vi "ColorText Facade.vi"(0 "Data In":T4, 2 "Display State In":T2, 3 "Container State":T3) -> (6 "Data Out":T4, 7 "Display State Out":T2, 8 "Action":T1)   [LabVIEW 2020, in "Code.xctl"]
uses:
  Code.xctl
  ColorText Data.ctl
  <vilib>/_xctls/Container State.ctl
  ColorText State.ctl
  <vilib>/_xctls/Action.ctl
  <vilib>/_xctls/XControlSupport.lvlib
panel:
  in  "Rows":string
  in  "Code":string
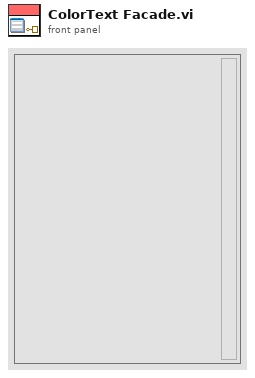
[diagram p1: front panel]
types:
  T1 = typedef "XControlSupport.lvlib/Action.ctl" = cluster{"Data Changed?":bool, "State Changed?":bool, "Action Name":string}
  T2 = typedef "Code.xctl/ColorText State.ctl" = cluster{"Numeric":dbl}
  T3 = typedef "XControlSupport.lvlib/Container State.ctl" = cluster{"Indicator?":bool, "Run Mode?":bool, " Refnum":refnum<vi>}
  T4 = typedef "Code.xctl/ColorText Data.ctl" = string
  T5 = cluster{"Code":refnum<vi>, "Panel":refnum<vi>, "Rows":refnum<vi>}
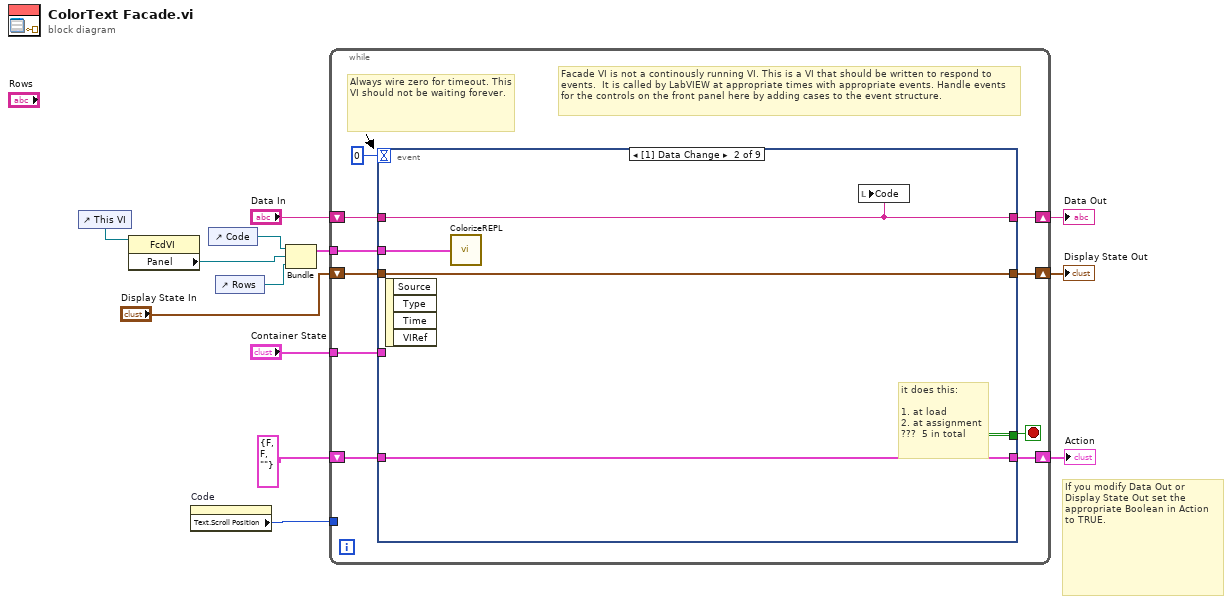
[diagram p0: block diagram]
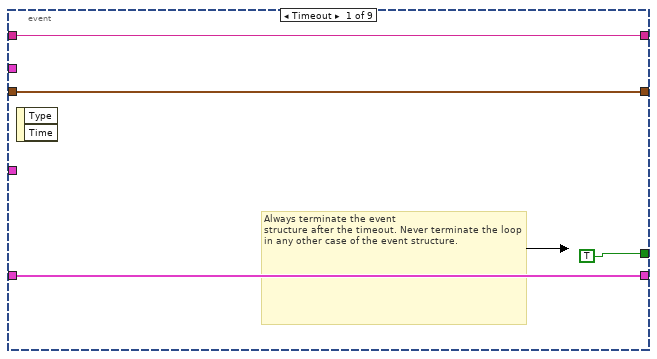
[diagram p2: hidden frame]
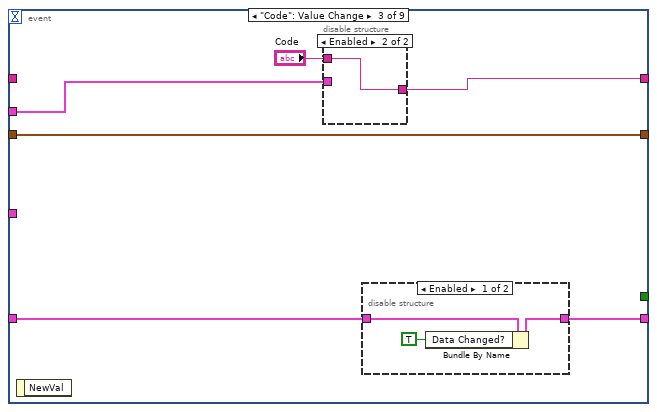
[diagram p3: hidden frame]
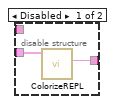
[diagram p4: hidden frame]
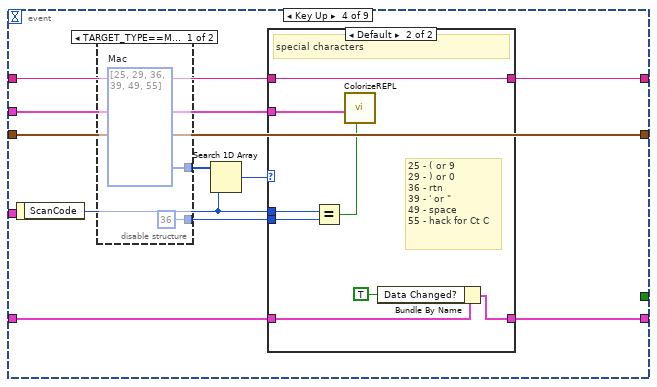
[diagram p6: hidden frame]
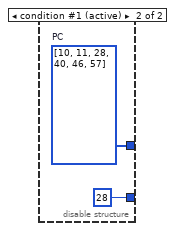
[diagram p7: hidden frame]
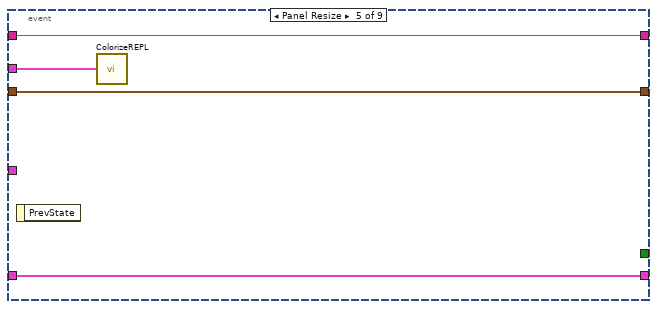
[diagram p9: hidden frame]
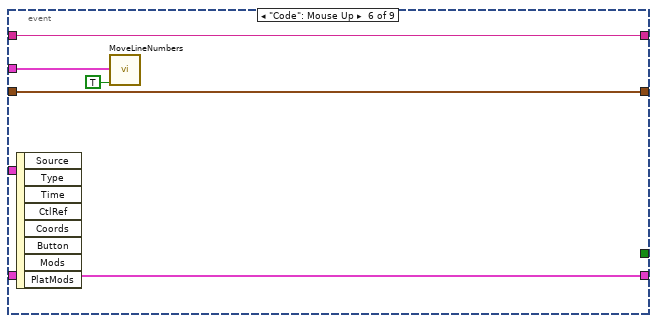
[diagram p10: hidden frame]
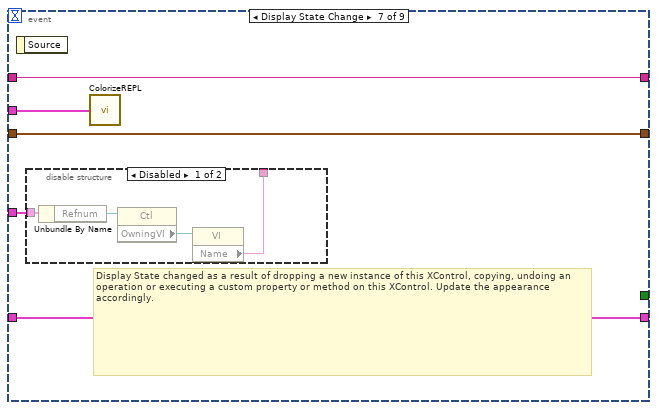
[diagram p11: hidden frame]
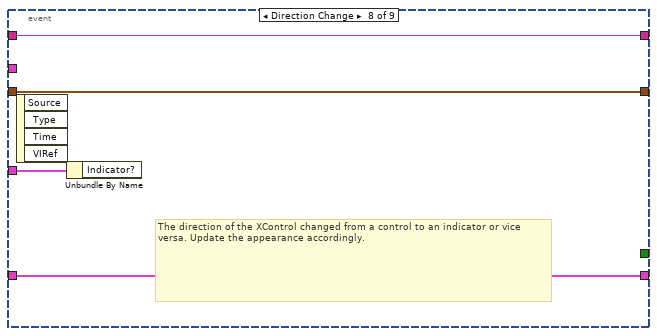
[diagram p13: hidden frame]
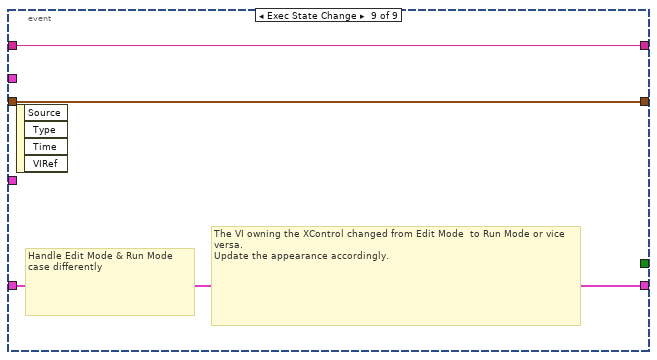
[diagram p14: hidden frame]
diagram:
  # "If you modify Data Out or\nDisplay State Out set the\nappropriate Boolean in Action\nto TRUE."
  n1 = control-ref of="This VI"() -> (w6:refnum<vi>)
  n2 = property class="FcdVI"(reference=w6) -> ("Panel"=w4:refnum<vi>)  [unwired: 1 in, 2 out]
  n3 = property on="Code" class="Str"() -> ("Text.Scroll Position"=w2:u32)  [unwired: 2 in, 2 out]
  n4 = control-ref of="Code"() -> (w3:refnum<vi>)
  n5 = control-ref of="Rows"() -> (w1:refnum<vi>)
  n6 = Bundle("Code"=w3, "Panel"=w4, "Rows"=w1) -> (w5:T5)  [unwired: 1 in]
  n7 = while {
    shift-right: [w22] -> w10
    shift-left: "Display State In" -> [w23]
    tunnel: "Container State" -> [w20]
    shift-right: [w14] -> w13
    shift-left: "Data In" -> [w19]
    shift-right: [w17] -> w8
    shift-left: T1 {"Data Changed?"=FALSE, "State Changed?"=FALSE, "Action Name"=""} ("Action") -> [w18]
    tunnel: w5 -> [w15]
    tunnel: w2 -> [_]
    stop <- w21 stop-if-true
    # "Facade VI is not a continously running VI. This is a VI that should be written to respond to events.  It is called by LabVIEW at appropriate times with appropriate events. Handle events for the controls on the front panel here by adding cases to the event structure."
    # "Always wire zero for timeout. This\nVI should not be waiting forever."
    n8 = event shown="[1] Data Change" {
      selector: _ -> [_ _ _ _ _ _ _ _ _]
      dyn-events: _ -> [_ _ _ _ _ _ _ _ _]
      timeout: 0 -> [_ _ _ _ _ _ _ _ _]
      tunnel: w23 -> [w25 w31 w37 w54 w72 w77 w82 w89 w93]
      tunnel: [w25 w31 w37 w54 w72 w77 w82 w89 w93] -> w22
      tunnel: [TRUE _ _ _ _ _ _ _ _] -> w21
      tunnel: w20 -> [_ _ _ _ _ _ w78 w90 _]
      tunnel: w19 -> [w24 w29 _ w51 w70 w74 w80 w87 w91]
      tunnel: [w26 w30 w35 w52 w69 w76 w81 w88 w92] -> w17
      tunnel: w18 -> [w26 w30 w36 w53 w69 w76 w81 w88 w92]
      tunnel: w15 -> [_ w28 w34 w50 w71 w75 w79 _ _]
      tunnel: [w24 w29 w33 w49 w70 w74 w80 w87 w91] -> w14
      event Timeout {
        # "Always terminate the event\nstructure after the timeout. Never terminate the loop in any other case of the event structure."
        n9 = event-data() -> ()  [unwired: 1 in, 2 out]
      }
      event Data Change {
        # "it does this:\n\n1. at load\n2. at assignment\n???  5 in total"
        n10 = event-data() -> ()  [unwired: 1 in, 4 out]
        n11 = call "ColorizeREPL.vi"("Refs"=w28) -> ()  [unwired: 9 in, 1 out]
        n12 = local write "Code"(w29) -> ()
      }
      event "Code": Value Change {
        n13 = event-data() -> ()  [unwired: 1 in, 1 out]
        n14 = disable-structure shown="Enabled" {
          disable-tunnel: w34 -> [w39 _]
          disable-tunnel: [w38 w40] -> w33
          disable-tunnel: "Code" -> [_ w40]
          frame Disabled {
            n15 = call "ColorizeREPL.vi"("Refs"=w39) -> ("Value"=w38:string)  [unwired: 9 in]
          }
          frame Enabled {
          }
        }
        n16 = disable-structure shown="Enabled" {
          disable-tunnel: w36 -> [w43 w44]
          disable-tunnel: [w42 w44] -> w35
          frame Enabled {
            n17 = Bundle By Name(cluster=w43, "Data Changed?"=TRUE) -> (w42:T1)
          }
          frame Disabled {
          }
        }
      }
      event Key Up {
        n18 = event-data() -> ("ScanCode"=w46:i16)  [unwired: 1 in]
        n19 = disable-structure shown="TARGET_TYPE==Mac, Default" {
          disable-tunnel: [w56 w58] -> w48
          disable-tunnel: [i16 36 ("y") i16 28 ("y")] -> w45
          frame condition #0 {
            w56 = i32[] [25, 29, 36, 39, 49, 55]  # Mac
          }
          frame condition #1 (active) {
            w58 = i32[] [10, 11, 28, 40, 46, 57]  # PC
          }
        }
        n20 = Search 1D Array(1D array=w48, element=w46) -> (index of element=w47:i32)  [unwired: 1 in]
        n21 = case shown="Default" w47 {
          tunnel: w53 -> [w60 w67]
          tunnel: [w60 w66] -> w52
          tunnel: w51 -> [w59 w64]
          tunnel: [w59 w64] -> w49
          tunnel: w50 -> [_ w65]
          tunnel: w46 -> [_ w62]
          tunnel: w45 -> [_ w61]
          frame -1 {
          }
          frame Default {
            # "25 - ( or 9\n29 - ) or 0\n36 - rtn\n39 - ' or \"\n49 - space\n55 - hack for Ct C"
            # "special characters"
            n22 = Equal?(x=w62, y=w61) -> (x = y?=w63:bool)
            n23 = call "ColorizeREPL.vi"("Refs"=w65, "Add Spaces?"=w63) -> ()  [unwired: 8 in, 1 out]
            n24 = Bundle By Name(cluster=w67, "Data Changed?"=TRUE) -> (w66:T1)
          }
        }
      }
      event Panel Resize {
        n25 = event-data() -> ()  [unwired: 1 in, 1 out]
        n26 = call "ColorizeREPL.vi"("Refs"=w71) -> ()  [unwired: 9 in, 1 out]
      }
      event "Code": Mouse Up {
        n27 = event-data() -> ()  [unwired: 1 in, 8 out]
        n28 = call "MoveLineNumbers.vi"("Force?"=TRUE, "Refs"=w75) -> ()  [unwired: 10 in]
      }
      event Display State Change {
        # "Display State changed as a result of dropping a new instance of this XControl, copying, undoing an operation or executing a custom property or method on this XControl. Update the appearance accordingly."
        n29 = event-data() -> ()  [unwired: 1 in, 1 out]
        n30 = disable-structure shown="Disabled" {
          disable-tunnel: w78 -> [w86 _]
          disable-tunnel: [w83 _] -> _
          frame Disabled {
            n31 = Unbundle By Name(w86) -> ("Refnum"=w85:refnum<vi>)
            n32 = property class="Ctl"(reference=w85) -> ("OwningVI"=w84:refnum<vi>)  [unwired: 1 in, 2 out]
            n33 = property class="VI"(reference=w84) -> ("Name"=w83:string)  [unwired: 1 in, 2 out]
          }
          frame Enabled {
          }
        }
        n34 = call "ColorizeREPL.vi"("Refs"=w79) -> ()  [unwired: 9 in, 1 out]
      }
      event Direction Change {
        # "The direction of the XControl changed from a control to an indicator or vice versa. Update the appearance accordingly."
        n35 = event-data() -> ()  [unwired: 1 in, 4 out]
        n36 = Unbundle By Name(w90) -> ()  [unwired: 1 out]
      }
      event Exec State Change {
        # "The VI owning the XControl changed from Edit Mode  to Run Mode or vice versa.\nUpdate the appearance accordingly."
        # "Handle Edit Mode & Run Mode\ncase differently"
        n37 = event-data() -> ()  [unwired: 1 in, 4 out]
      }
    }
  }
  "Display State Out" <- w10
  "Data Out" <- w13
  "Action" <- w8
